vi "IMAQ FPGA Pixel Bus to FIFO U16x8.vi"(8 "Input Valid":bool=TRUE, 10 "Destination Image FIFO":refnum<k21>, 11 "Pixel Bus In":T1={"Pixel Data"=[0, 0, 0, 0, 0, 0, 0, 0], "DV"=[FALSE, FALSE, FALSE, FALSE, FALSE, FALSE, FALSE, FALSE], "EOL"=FALSE, "EOI"=FALSE, "Data Type"=enum."U16 x 8"}) -> (4 "Ready For Input":bool)   [LabVIEW 2020, in "NI_VDM_FPGA_Basics.lvlib"]
doc: "Writes valid Pixel Data in the Pixel Bus cluster to the specified FIFO. If the FIFO is full, the Ready for Input terminal returns FALSE during that cycle."
uses:
  <vilib>/visionFPGA/NI_VDM_FPGA_Basics.lvlib
  <vilib>/rvi/DataTransferAndStorage/Container/XNode/niFpgaContainer.xnode
  <vilib>/rvi/FIFO/Fifo_Resource/niFpgaFifoEmulationRefInMultiElement.vi
  <vilib>/visionFPGA/Controls/IMAQ FPGA Pixel Bus u16x8.ctl
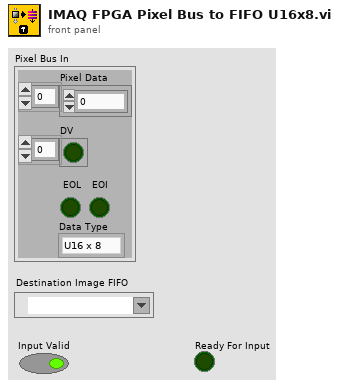
[diagram p1: front panel]
types:
  T1 = typedef "IMAQ FPGA Pixel Bus u16x8.ctl" = cluster{"Pixel Data":u16[], "DV":bool[], "EOL":bool, "EOI":bool, "Data Type":enum16{"U16 x 8"}}
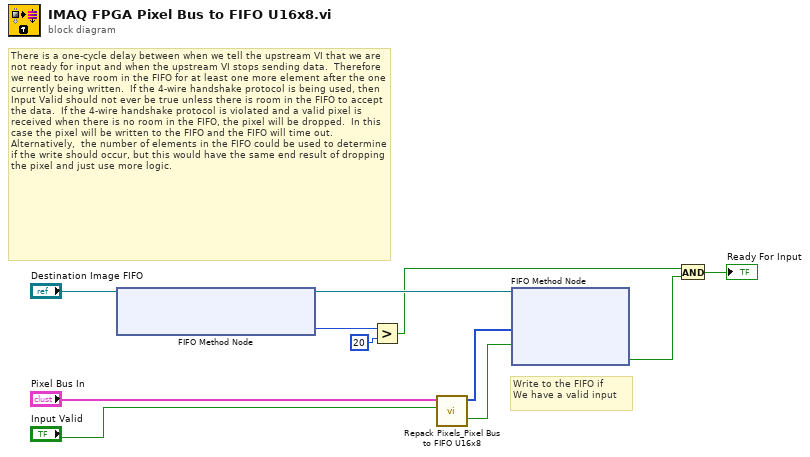
[diagram p0: block diagram]
diagram:
  # "There is a one-cycle delay between when we tell the upstream VI that we are not ready for input and when the upstream VI stops sending data.  Therefore we need to have room in the FIFO for at least one more element after the one currently being written.  If the 4-wire handshake protocol is being used, then Input Valid should not ever be true unless there is room in the FIFO to accept the data.  If the 4-wire handshake protocol is violated and a valid pixel is received when there is no room in the FIFO, the pixel will be dropped.  In this case the pixel will be written to the FIFO and the FIFO will time out.  Alternatively,  the number of elements in the FIFO could be used to determine if the write should occur, but this would have the same end result of dropping the pixel and just use more logic."
  # "Write to the FIFO if \nWe have a valid input"
  n1 = xnode ("FIFO Method Node")("FIFO In"="Destination Image FIFO") -> ("Number of Elements to Write"=w5:u32, "FIFO Out"=w6:refnum<k21>)
  n2 = Greater?(x=w5, y=u32 20) -> (0:w2:bool)
  n3 = call <vilib>:"Repack Pixels_Pixel Bus to FIFO U16x8.vi"("Input Valid"="Input Valid", "Pixel Bus In"="Pixel Bus In") -> ("Output Valid"=w4:bool, "output array"=w9:u16[])  [unwired: 8 in]
  n4 = xnode ("FIFO Method Node")("Element"=w9, "Input Valid"=w4, "FIFO In"=w6) -> ("Ready for Input"=w3:bool)  [unwired: 1 out]
  n5 = And(x=w2, y=w3) -> (x .and. y?=→"Ready For Input":bool)
